vi "Open Recording File1.vi"(8 "error in (no error)":errorcluster, 11 "AcquireTraces In":refnum<class "AcquireTraces.lvclass">) -> (0 "error out":errorcluster, 3 "AcquireTraces Out":refnum<class "AcquireTraces.lvclass">)   [LabVIEW 2011, in "AcquireTraces.lvclass"]
uses:
  AcquireTraces/AcquireTraces.lvclass
  AcquireTraces/AcquireTraces.lvclass/AcquireTraces.ctl
  HDF5Tools/LabView/Create Dataset 2D Integer.vi
  HDF5Tools/LabView/HDF5Tools.lvlib
  Program Files/National Instruments/LabVIEW 2011/resource/objmgr/daqmx.rc
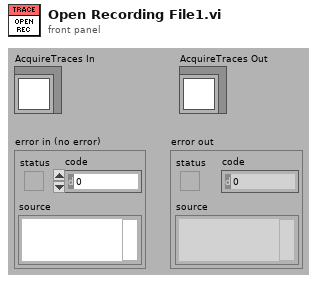
[diagram p1: front panel]
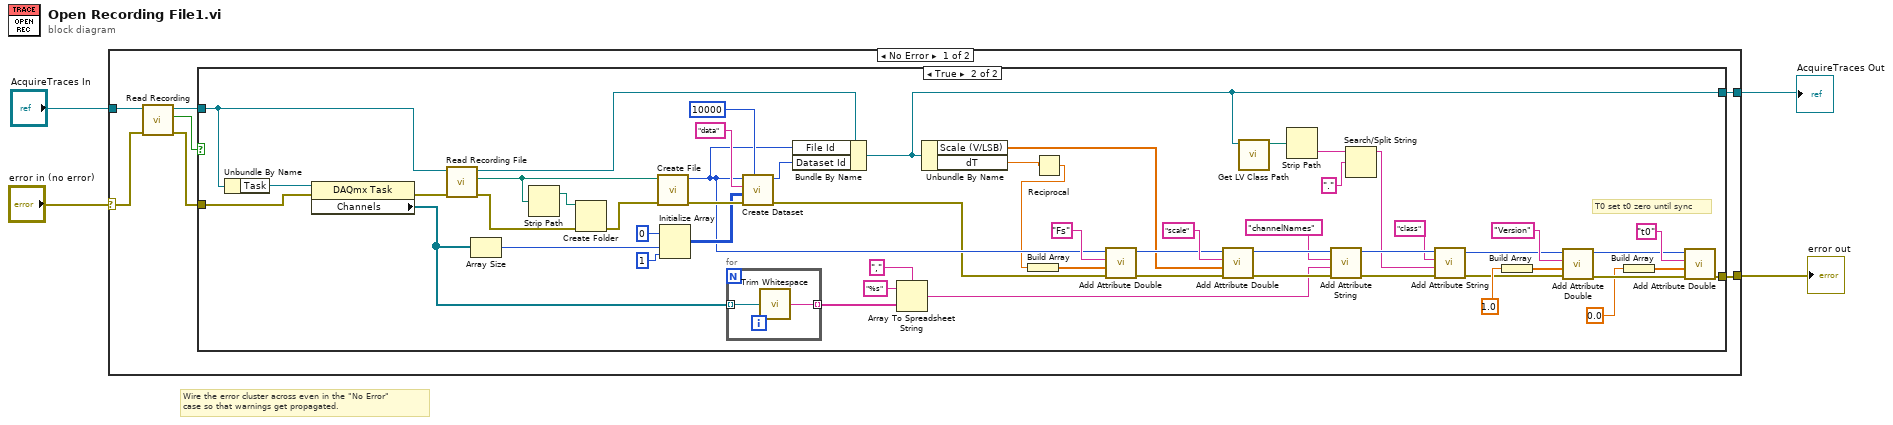
[diagram p0: block diagram]
diagram:
  # "Wire the error cluster across even in the \"No Error\"\ncase so that warnings get propagated."
  n1 = case shown="No Error" "error in (no error)" {
    selector: "error in (no error)" -> [w6 w71]
    tunnel: [w10 w71] -> w3
    tunnel: [w11 w70] -> w2
    tunnel: "AcquireTraces In" -> [w9 w70]
    frame No Error {
      n2 = call-dynamic "Read Recording.vi"("error in (no error)"=w6, "AcquireTraces in"=w9) -> ("error out"=w5:errorcluster, "Recording"=w7:bool, "AcquireTraces out"=w8:refnum<class "AcquireTraces.lvclass">)  [unwired: 7 in]
      n3 = case shown="True" w7 {
        tunnel: w8 -> [w13 w59]
        tunnel: w5 -> [w12 w45]
        tunnel: [w13 w35] -> w11
        tunnel: [w12 w20] -> w10
        frame False {
        }
        frame True {
          # "T0 set t0 zero until sync"
          n4 = Unbundle By Name(w59) -> ("Task"=w46:refnum<k21>)
          n5 = property class="DAQmx Task"(reference=w46, error in=w45) -> (error out=w43:errorcluster, "Channels"=w40:refnum<k21>[])  [unwired: 1 out]
          n6 = call-dynamic "Read Recording File.vi"("error in (no error)"=w43, "AcquistionObject in"=w59) -> ("error out"=w15:errorcluster, "Recording File"=w16:path, "AcquistionObject out"=w60:refnum<class "AcquireTraces.lvclass">)  [unwired: 7 in]
          n7 = Array Size(array=w40) -> (size(s)=w44:i32)
          n8 = Strip Path(path=w16) -> (stripped path=w17:path)  [unwired: 1 out]
          n9 = Create Folder(path (use dialog)=w17, error in=w15) -> (error out=w14:errorcluster)  [unwired: 1 in, 2 out]
          n10 = call "Create File.vi"("Error in"=w14, "File Name"=w16) -> ("Error out"=w67:errorcluster, "file_id"=w42:i32)  [unwired: 6 in]
          n11 = Initialize Array(0, w44, 1 ("dimension size")) -> (w62:i32[][])
          n12 = for {
            tunnel: w40 -> [w68] mode=indexing
            tunnel: [w69] -> w52 mode=indexing
            n13 = call <vilib>:"Trim Whitespace.vi"("string"=w68) -> ("trimmed string"=w69:string)  [unwired: 1 in]
          }
          n14 = call-poly "Create Dataset.vi"("Chunk size"=10000, "error in (no error)"=w67, "Datatype"=w62, "Dataset name"="data", "Location id in"=w42) -> ("error out"=w41:errorcluster, "Dataset id"=w61:i32)  [unwired: 5 in]
          n15 = Bundle By Name(cluster=w60, "File Id"=w42, "Dataset Id"=w61) -> (w35:refnum<class "AcquireTraces.lvclass">)
          n16 = Array To Spreadsheet String(delimiter (Tab)=",", array=w52, 3:"%s" ("format string")) -> (spreadsheet string=w47:string)
          n17 = Unbundle By Name(w35) -> ("Scale (V/LSB)"=w18:dbl[], "dT"=w26:dbl)
          n18 = Reciprocal(x=w26) -> (1/x=w25:dbl)
          n19 = Build Array(w25) -> (w57:dbl[])
          n20 = call "Add Attribute Double.vi"("error in (no error)"=w41, "data"=w57, "Attribute name"="Fs", "loc_id"=w42) -> ("error out"=w56:errorcluster, "loc_id_out"=w49:i32)  [unwired: 6 in]
          n21 = call "Add Attribute Double.vi"("error in (no error)"=w56, "data"=w18, "Attribute name"="scale", "loc_id"=w49) -> ("error out"=w51:errorcluster, "loc_id_out"=w50:i32)  [unwired: 6 in]
          n22 = call <vilib>:"Get LV Class Path.vi"("object"=w35) -> ("class path"=w38:path)  [unwired: 9 in, 1 out]
          n23 = Strip Path(path=w38) -> (name=w37:string)  [unwired: 1 out]
          n24 = call "Add Attribute String.vi"("error in (no error)"=w51, "Attribute data"=w47, "Attribute name"="channelNames", "loc_id"=w50) -> ("error out"=w33:errorcluster, "loc_id_out"=w39:i32)  [unwired: 6 in]
          n25 = Search/Split String(string=w37, search string/char (-)=".") -> (substring before match=w32:string)  [unwired: 1 in, 2 out]
          n26 = call "Add Attribute String.vi"("error in (no error)"=w33, "Attribute data"=w32, "Attribute name"="class", "loc_id"=w39) -> ("error out"=w29:errorcluster, "loc_id_out"=w27:i32)  [unwired: 6 in]
          n27 = Build Array(1.0) -> (w28:dbl[])
          n28 = call "Add Attribute Double.vi"("error in (no error)"=w29, "data"=w28, "Attribute name"="Version", "loc_id"=w27) -> ("error out"=w22:errorcluster, "loc_id_out"=w21:i32)  [unwired: 6 in]
          n29 = Build Array(0.0 ("element")) -> (w23:dbl[])
          n30 = call "Add Attribute Double.vi"("error in (no error)"=w22, "data"=w23, "Attribute name"="t0", "loc_id"=w21) -> ("error out"=w20:errorcluster)  [unwired: 6 in, 1 out]
        }
      }
    }
    frame Error {
    }
  }
  "error out" <- w3
  "AcquireTraces Out" <- w2
